vi "subvi_encoder_update.vi"(4 "Position Reset":bool, 6 "Tick'":i32, 7 "A":bool, 9 "B'":bool, 10 "A'":bool, 11 "B":bool) -> (3 "Tick":i32)   [LabVIEW 2019]
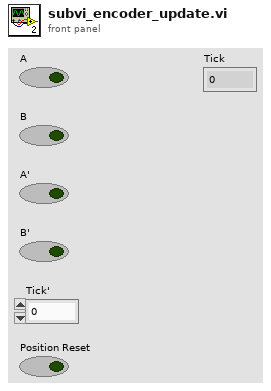
[diagram p1: front panel]
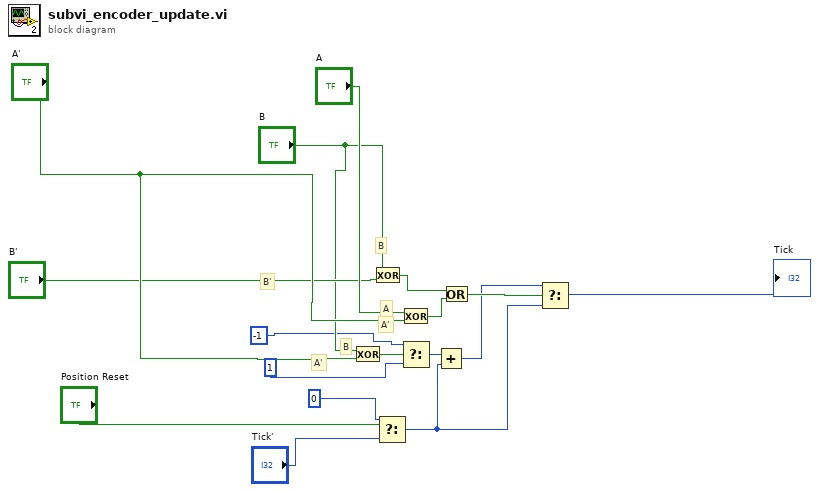
[diagram p0: block diagram]
diagram:
  # "B'"
  # "A'"
  # "B"
  # "A'"
  # "A"
  # "B"
  n1 = Exclusive Or(1:"A'", 2:"B") -> (0:w11:bool)
  n2 = Exclusive Or(1:"B'", 2:"B") -> (0:w10:bool)
  n3 = Select(t=0 ("32 bit"), s="Position Reset", f="Tick'") -> (s? t:f=w4:i32)
  n4 = Exclusive Or(1:"A'", 2:"A") -> (0:w9:bool)
  n5 = Select(t=-1 ("32 bit"), s=w11, f=1 ("32 bit")) -> (s? t:f=w6:i32)
  n6 = Add(x=w6, y=w4) -> (x+y=w2:i32)
  n7 = Or(x=w10, y=w9) -> (x .or. y?=w12:bool)
  n8 = Select(t=w2, s=w12, f=w4) -> (s? t:f=→"Tick":i32)
